vi "Voice_coil_control.vi"() -> ()   [LabVIEW 2020]
uses:
  <vilib>/DAQmx/write.llb/DAQmx Write (Analog DBL 1Chan 1Samp).vi
  <vilib>/DAQmx/create/channels.llb/DAQmx Create Channel (AO-Voltage-Basic).vi
  <vilib>/DAQmx/miscellaneous.llb/DAQmx Fill In Error Info.vi
panel:
  in  "Manual voice coil voltage":bool
  in  "stop":bool
  in  "error in":errorcluster
  in  "Stop Button":bool
  in  "Voice coil voltage slider":dbl(slide) min=-0.6 max=0.6 scale=-0.6..0.6
  in  "Voice coil voltage input":dbl min=-0.6 max=0.6 format="%#_3g"
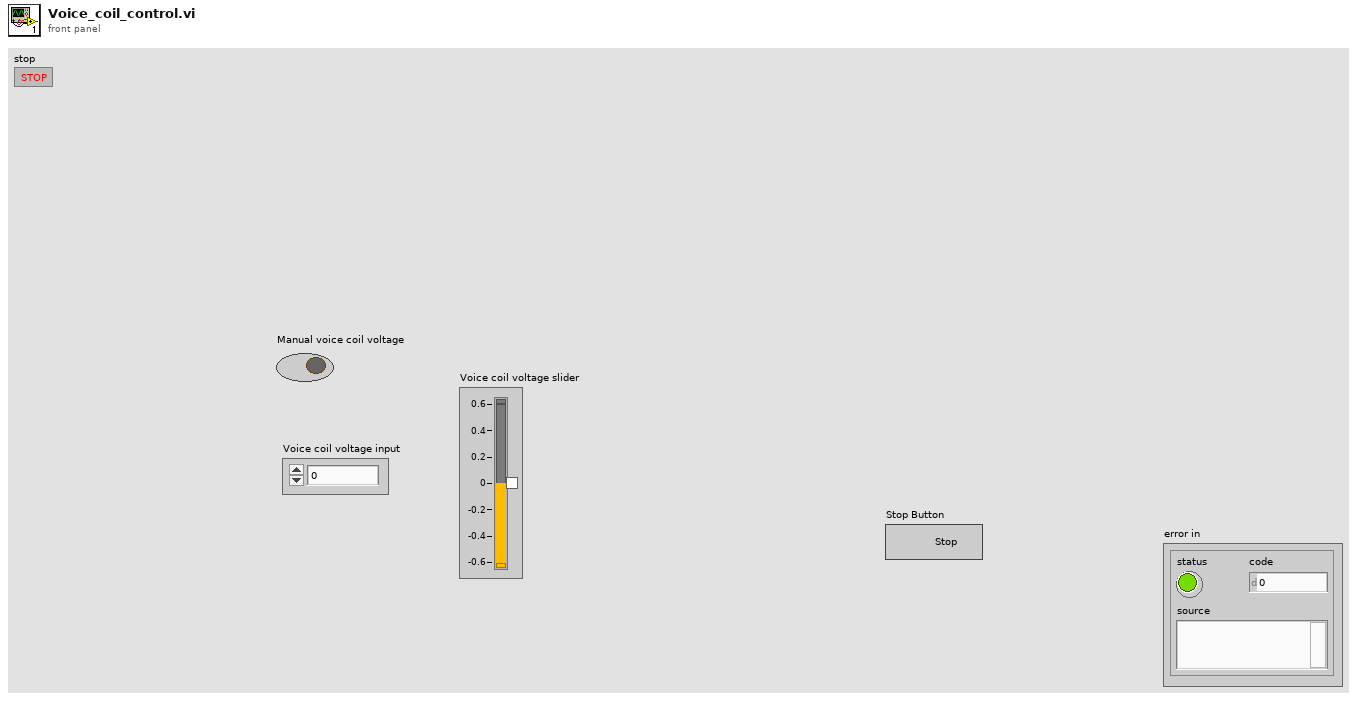
[diagram p1: front panel]
types:
  T1 = enum8{"Enabled", "Disabled", "Disabled and Grayed Out"}
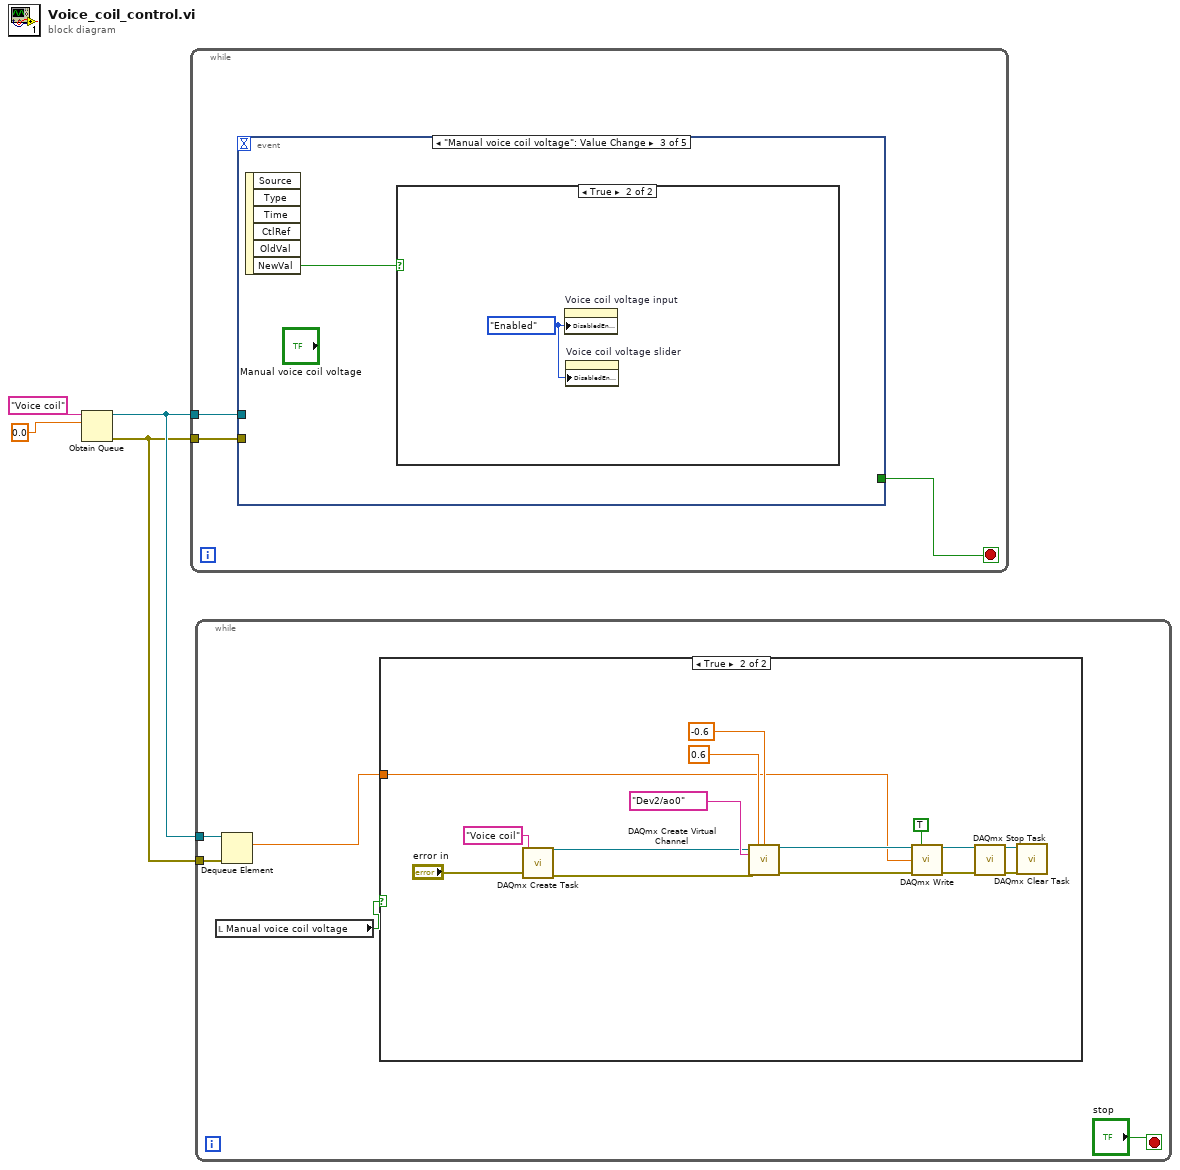
[diagram p0: block diagram]
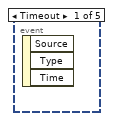
[diagram p3: hidden frame]
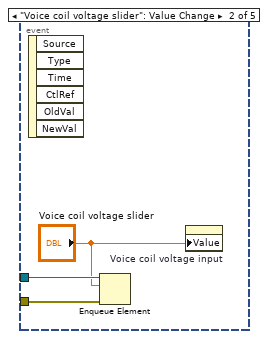
[diagram p4: hidden frame]
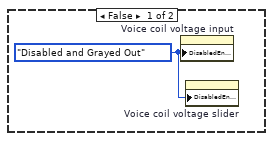
[diagram p5: hidden frame]
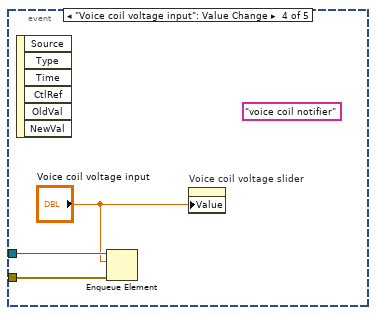
[diagram p6: hidden frame]
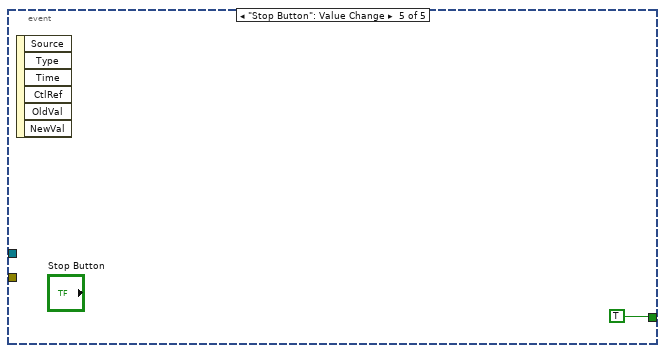
[diagram p7: hidden frame]
diagram:
  n1 = Obtain Queue(name (unnamed)="Voice coil", element data type=0.0) -> (queue out=w2:refnum<queue>, error out=w1:errorcluster)  [unwired: 3 in, 1 out]
  n2 = while {
    tunnel: w2 -> [w7]
    tunnel: w1 -> [w6]
    stop <- w5 stop-if-true
    n3 = event shown="[2] \"Manual voice coil voltage\": Value Change" {
      selector: _ -> [_ _ _ _ _]
      dyn-events: _ -> [_ _ _ _ _]
      timeout: _ -> [_ _ _ _ _]
      tunnel: [_ _ _ _ TRUE] -> w5
      tunnel: w7 -> [_ w10 _ w16 _]
      tunnel: w6 -> [_ w9 _ w15 _]
      event Timeout {
        n4 = event-data() -> ()  [unwired: 1 in, 3 out]
      }
      event "Voice coil voltage slider": Value Change {
        n5 = event-data() -> ()  [unwired: 1 in, 6 out]
        n6 = Enqueue Element(queue=w10, element="Voice coil voltage slider", error in (no error)=w9) -> ()  [unwired: 1 in, 3 out]
        n7 = property on="Voice coil voltage input" class="DigNum (strict)"("Value"="Voice coil voltage slider") -> ()  [unwired: 2 in, 2 out]
      }
      event "Manual voice coil voltage": Value Change {
        n8 = event-data() -> ("NewVal"=w11:bool)  [unwired: 1 in, 5 out]
        n9 = case shown="True" w11 {
          frame False {
            w12 = T1."Disabled and Grayed Out" ("Disabled")
            n10 = property on="Voice coil voltage input" class="DigNum (strict)"("DisabledEnum"=w12) -> ()  [unwired: 2 in, 2 out]
            n11 = property on="Voice coil voltage slider" class="Slide (strict)"("DisabledEnum"=w12) -> ()  [unwired: 2 in, 2 out]
          }
          frame True {
            w13 = T1."Enabled" ("Disabled")
            n12 = property on="Voice coil voltage input" class="DigNum (strict)"("DisabledEnum"=w13) -> ()  [unwired: 2 in, 2 out]
            n13 = property on="Voice coil voltage slider" class="Slide (strict)"("DisabledEnum"=w13) -> ()  [unwired: 2 in, 2 out]
          }
        }
      }
      event "Voice coil voltage input": Value Change {
        (unwired) "voice coil notifier" ("name (unnamed)")
        n14 = event-data() -> ()  [unwired: 1 in, 6 out]
        n15 = Enqueue Element(queue=w16, element="Voice coil voltage input", error in (no error)=w15) -> ()  [unwired: 1 in, 3 out]
        n16 = property on="Voice coil voltage slider" class="Slide (strict)"("Value"="Voice coil voltage input") -> ()  [unwired: 2 in, 2 out]
      }
      event "Stop Button": Value Change {
        n17 = event-data() -> ()  [unwired: 1 in, 6 out]
      }
    }
  }
  n18 = while {
    tunnel: w2 -> [w22]
    tunnel: w1 -> [w21]
    stop <- "stop" stop-if-true
    n19 = local read "Manual voice coil voltage"() -> (w18:bool)
    n20 = Dequeue Element(queue=w22, error in (no error)=w21) -> (element=w20:dbl)  [unwired: 1 in, 3 out]
    n21 = case shown="True" w18 {
      tunnel: w20 -> [_ w23]
      frame False {
      }
      frame True {
        n22 = call <vilib>:"DAQmx Create Task.vi"("new task name"="Voice coil", "error in"="error in") -> ("task out"=w35:refnum<k21>, "error out"=w34:errorcluster)  [unwired: 12 in]
        n23 = call-poly <vilib>:"DAQmx Create Virtual Channel.vi"("task in"=w35, "maximum value"=0.6, "minimum value"=-0.6, "physical channels"=tag "Dev2/ao0", "error in"=w34) -> ("task out"=w30:refnum<k21>, "error out"=w29:errorcluster)  [unwired: 9 in]
        n24 = call-poly <vilib>:"DAQmx Write.vi"("task/channels in"=w30, "auto start"=TRUE, "data"=w23, "error in"=w29) -> ("task out"=w25:refnum<k21>, "error out"=w24:errorcluster)  [unwired: 9 in, 1 out]
        n25 = call <vilib>:"DAQmx Stop Task.vi"("task/channels in"=w25, "error in"=w24) -> ("task out"=w26:refnum<k21>, "error out"=w27:errorcluster)  [unwired: 12 in]
        n26 = call <vilib>:"DAQmx Clear Task.vi"("task in"=w26, "error in"=w27) -> ()  [unwired: 13 in, 1 out]
      }
    }
  }
